vi "DemoTrigApp_SUB_SelectDOCh_Panel.vi"() -> (1 "Cancel":bool, 2 "NegPos":enum16{"Neg", "Pos"}(ring), 3 "DO ch":tag)   [LabVIEW 2012]
panel:
  in  "Btn NegPos":bool
  out "Select NegPos":u16(ring) caption="Trigger Type" items=["Neg", "Pos"]
  in  "Btn Cancel":bool
  in  "Btn OK":bool
  in  "DO ch":tag="Dev1/port0/line0" caption="Select Digital Output Channel"
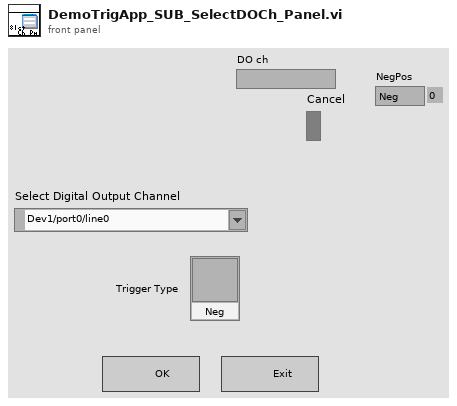
[diagram p1: front panel]
types:
  T1 = enum8{"Enabled", "Disabled", "Disabled and Grayed Out"}
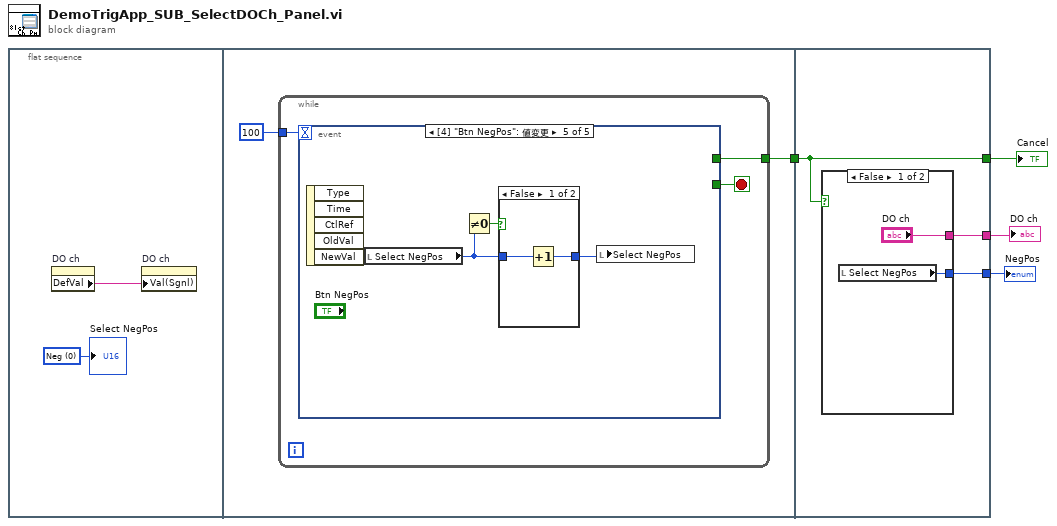
[diagram p0: block diagram]
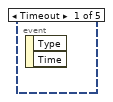
[diagram p2: hidden frame]
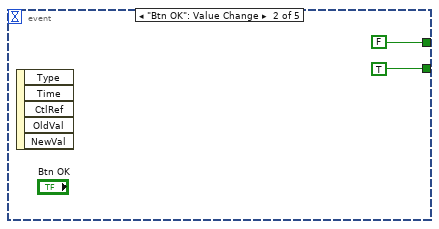
[diagram p3: hidden frame]
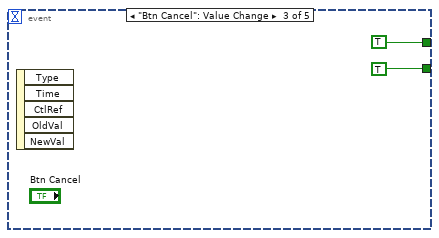
[diagram p4: hidden frame]
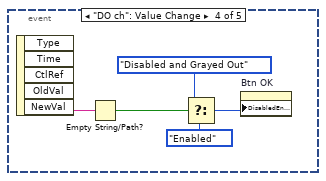
[diagram p5: hidden frame]
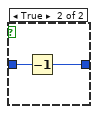
[diagram p6: hidden frame]
diagram:
  n1 = flat-sequence {
    tunnel: [w7] -> w4
    tunnel: w4 -> [w30]
    tunnel: [w30] -> w3
    tunnel: [w29] -> w2
    tunnel: [w28] -> w1
    frame #0 {
      w5 = u16 0 items=["Neg", "Pos"]
      n2 = property on="DO ch" class="DAQmxName"() -> ("DefVal"=w6:string)  [unwired: 2 in, 2 out]
      n3 = property on="DO ch" class="DAQmxName"("Val(Sgnl)"=w6) -> ()  [unwired: 2 in, 2 out]
      "Select NegPos" <- w5
    }
    frame #1 {
      n4 = while {
        tunnel: 100 -> [w11]
        tunnel: [w9] -> w7
        stop <- w10 stop-if-true
        n5 = event shown="[4] \"Btn NegPos\": 値変更" {
          selector: _ -> [_ _ _ _ _]
          dyn-events: _ -> [_ _ _ _ _]
          timeout: w11 -> [_ _ _ _ _]
          tunnel: [_ TRUE TRUE _ _] -> w10
          tunnel: [_ FALSE TRUE _ _] -> w9
          event Timeout {
            n6 = event-data() -> ()  [unwired: 1 in, 2 out]
          }
          event "Btn OK": Value Change {
            n7 = event-data() -> ()  [unwired: 1 in, 5 out]
          }
          event "Btn Cancel": Value Change {
            n8 = event-data() -> ()  [unwired: 1 in, 5 out]
          }
          event "DO ch": Value Change {
            n9 = event-data() -> ("NewVal"=w20:tag)  [unwired: 1 in, 4 out]
            n10 = Empty String/Path?(string/path=w20) -> (empty?=w19:bool)
            n11 = Select(t=T1."Disabled and Grayed Out", s=w19, f=T1."Enabled") -> (s? t:f=w16:T1)
            n12 = property on="Btn OK" class="Bool"("DisabledEnum"=w16) -> ()  [unwired: 2 in, 2 out]
          }
          event "Btn NegPos": Value Change {
            n13 = event-data() -> ()  [unwired: 1 in, 5 out]
            n14 = local read "Select NegPos"() -> (w21:u16)
            n15 = Not Equal To 0?(x=w21) -> (x != 0?=w23:bool)
            n16 = case shown="FALSE" w23 {
              tunnel: w21 -> [w25 w27]
              tunnel: [w24 w26] -> w22
              frame False {
                n17 = Increment(x=w25) -> (x+1=w24:u16)
              }
              frame True {
                n18 = Decrement(x=w27) -> (x-1=w26:u16)
              }
            }
            n19 = local write "Select NegPos"(w22) -> ()
          }
        }
      }
    }
    frame #2 {
      n20 = case shown="FALSE" w30 {
        tunnel: ["DO ch" _] -> w29
        tunnel: [w31 _] -> w28
        frame False {
          n21 = local read "Select NegPos"() -> (w31:u16)
        }
        frame True {
        }
      }
    }
  }
  "Cancel" <- w3
  "DO ch" <- w2
  "NegPos" <- w1
